vi "Get Name.vi"(7 "Unique ID":string, 8 "error in (no error)":errorcluster, 11 "Test Executive in":refnum<class "Test Executive.lvclass">) -> (0 "error out":errorcluster, 1 "Tag":i32, 2 "Name":string, 3 "Test Executive out":refnum<class "Test Executive.lvclass">, 4 "Class":string)   [LabVIEW 2019, in "Test Executive.lvlib" / "Test Executive.lvclass"]
uses:
  <vilib>/gpm_packages/@cs/test-executive/Source/Test Executive/TestExecutive/Test Executive.lvclass
  <vilib>/gpm_packages/@cs/test-executive/Source/Test Executive/TestExecutive/Test Executive.lvclass/Test Executive.ctl
  <vilib>/gpm_packages/@cs/linked-list/Source/Linked List/Linked List Ref/Linked List Ref.lvclass
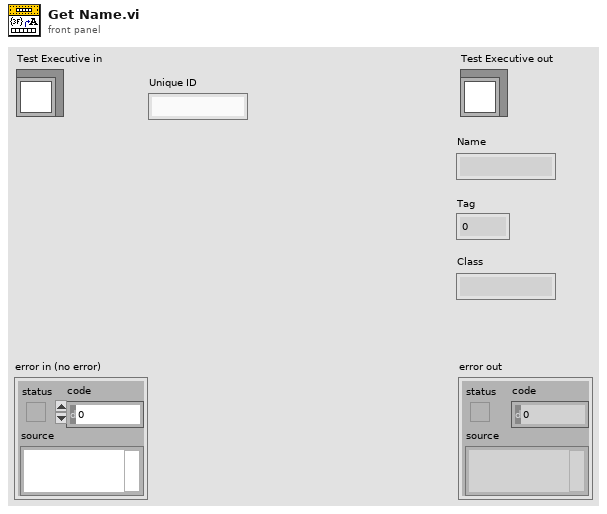
[diagram p1: front panel]
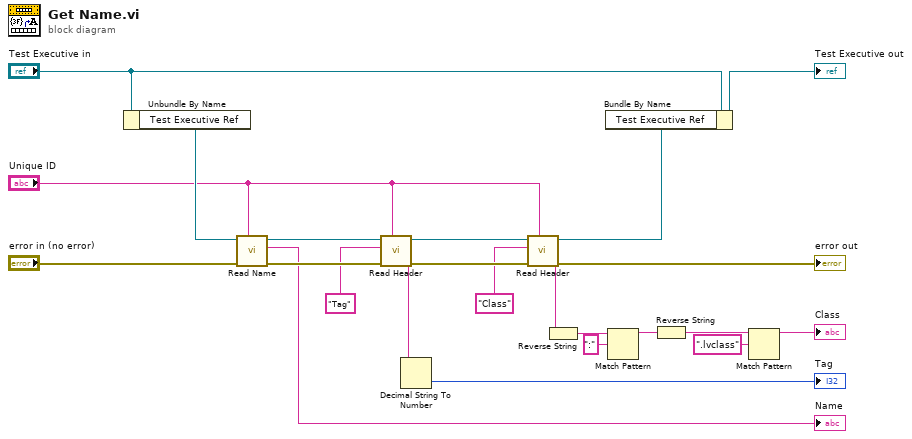
[diagram p0: block diagram]
diagram:
  n1 = Unbundle By Name("Test Executive in") -> ("Test Executive Ref"=w23:refnum<data-value>)
  n2 = call <vilib>:"Read Name.vi"("Linked List ID"="Unique ID", "error in (no error)"="error in (no error)", "Linked List Ref"=w23) -> ("error out"=w18:errorcluster, "Header Value"=→"Name":string, "Linked List Ref out"=w21:refnum<data-value>)  [unwired: 6 in]
  n3 = call <vilib>:"Read Header.vi"("Linked List ID"="Unique ID", "error in (no error)"=w18, "Header Name"="Tag" ("String"), "Linked List Ref"=w21) -> ("error out"=w17:errorcluster, "Header Value"=w9:string, "Linked List Ref out"=w20:refnum<data-value>)  [unwired: 4 in, 1 out]
  n4 = Decimal String To Number(string=w9) -> (number=→"Tag":i32)  [unwired: 2 in, 1 out]
  n5 = call <vilib>:"Read Header.vi"("Linked List ID"="Unique ID", "error in (no error)"=w17, "Header Name"="Class" ("String"), "Linked List Ref"=w20) -> ("error out"=→"error out":errorcluster, "Header Value"=w2:string, "Linked List Ref out"=w14:refnum<data-value>)  [unwired: 4 in, 1 out]
  n6 = Reverse String(1:w2) -> (0:w7:string)
  n7 = Bundle By Name(cluster="Test Executive in", "Test Executive Ref"=w14) -> (→"Test Executive out":refnum<class "Test Executive.lvclass">)
  n8 = Match Pattern(string=w7, regular expression=":") -> (before substring=w5:string)  [unwired: 1 in, 3 out]
  n9 = Reverse String(1:w5) -> (0:w4:string)
  n10 = Match Pattern(string=w4, regular expression=".lvclass") -> (before substring=→"Class":string)  [unwired: 1 in, 3 out]
